vi "MenuItem.vi"(7 "Selection Type":refnum<class "MGI_SelectionType.lvclass"> caption="Selection Type (Click)", 10 "error in (no error)":errorcluster, 11 "Text":string) -> (2 "error out":errorcluster, 3 "MenuItem":refnum<data-value>)   [LabVIEW 2016, in "MGI_MenuItem.lvclass"]
doc: "MenuItem Constructor. Each MenuItem will show up in the menu with the text defined. If Selection Type is left unwired, a \"click\" message is sent ever time the item is clicked.\n\nUse a Property Node to access the following properties:\nClick By Default\nFull Tag\nSelection Type\nSub-Menus\nTag\nText\n\nAuthored by Derek E. Trepanier\nsupport@mooregoodideas.com\nwww.mooregoodideas.com\n\nCopyright (c) 2012, Moore Good Ideas, Inc.\n\nAll rights reserved.\n\nRedistribution and use in source and binary forms, with or without modification, are permitted provided that the following conditions are met:\n\n * Redistributions of source code must retain the above copyright notice, this list of conditions and the following disclaimer.\n * Redistributions in binary form must reproduce the above copyright notice, this list of conditions and the following disclaimer in the documentation and/or other materials provided with the distribution.\n * Neither the name of Moore Good Ideas, Inc. nor the names of its contributors may be used to endorse or promote products derived from this software without specific prior written permission.\n\nTHIS SOFTWARE IS PROVIDED BY THE COPYRIGHT HOLDERS AND CONTRIBUTORS \"AS IS\" AND ANY EXPRESS OR IMPLIED WARRANTIES, INCLUDING, BUT NOT LIMITED TO, THE IMPLIED WARRANTIES OF MERCHANTABILITY AND FITNESS FOR A PARTICULAR PURPOSE ARE DISCLAIMED. IN NO EVENT SHALL THE COPYRIGHT OWNER OR CONTRIBUTORS BE LIABLE FOR ANY DIRECT, INDIRECT, INCIDENTAL, SPECIAL, EXEMPLARY, OR CONSEQUENTIAL DAMAGES (INCLUDING, BUT NOT LIMITED TO, PROCUREMENT OF SUBSTITUTE GOODS OR SERVICES; LOSS OF USE, DATA, OR PROFITS; OR BUSINESS INTERRUPTION) HOWEVER CAUSED AND ON ANY THEORY OF LIABILITY, WHETHER IN CONTRACT, STRICT LIABILITY, OR TORT (INCLUDING NEGLIGENCE OR OTHERWISE) ARISING IN ANY WAY OUT OF THE USE OF THIS SOFTWARE, EVEN IF ADVISED OF THE POSSIBILITY OF SUCH DAMAGE."
uses:
  <userlib>/_MGI/Menu Building/MenuItem/MGI_MenuItem.lvclass
  <userlib>/_MGI/Menu Building/SelectionType/MGI_SelectionType.lvclass
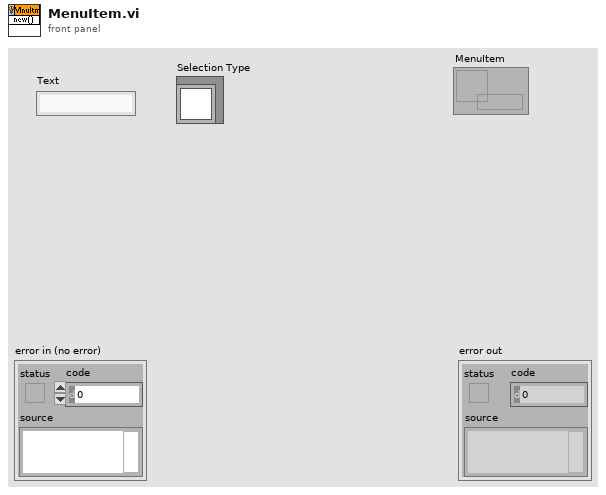
[diagram p1: front panel]
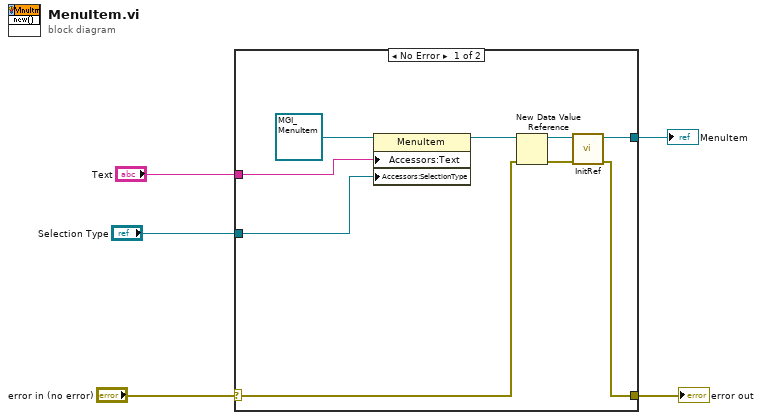
[diagram p0: block diagram]
diagram:
  n1 = case shown="No Error" "error in (no error)" {
    selector: "error in (no error)" -> [w13 w15]
    tunnel: [w6 w15] -> w4
    tunnel: [w8 _] -> w3
    tunnel: "Text" -> [w11 _]
    tunnel: "Selection Type" -> [w10 _]
    frame No Error {
      n2 = property class="MenuItem"(reference=refnum<class "MGI_MenuItem.lvclass"> refnum ("MenuItem out"), "Accessors:Text"=w11, "Accessors:SelectionType"=w10) -> (reference out=w12:refnum<class "MGI_MenuItem.lvclass">)  [unwired: 1 in, 1 out]
      n3 = New Data Value Reference(data value=w12, error in=w13) -> (data value reference=w9:refnum<data-value>, error out=w7:errorcluster)
      n4 = call <userlib>:"InitRef.vi"("error in (no error)"=w7, "MenuItem in"=w9) -> ("error out"=w6:errorcluster, "MenuItem out"=w8:refnum<data-value>)  [unwired: 8 in]
    }
    frame Error {
    }
  }
  "error out" <- w4
  "MenuItem" <- w3
